vi "Data Access.vi"(8 "error in (no error)":errorcluster, 10 "Data Access Handler":refnum<class "Data Access Handler.lvclass">, 11 "Multi Instrument Batch Msg in":refnum<class "Multi Instrument Batch Msg.lvclass">) -> (0 "error out":errorcluster, 3 "Multi Instrument Batch Msg out":refnum<class "Multi Instrument Batch Msg.lvclass">)   [LabVIEW 2020, in "Instrument Handler.lvlib" / "Multi Instrument Batch Msg.lvclass"]
doc: "Expose class private data to the front panel while letting the Data Access Handler class act on the data."
uses:
  Multi Instrument Batch Msg.lvclass
  C:/Current projects/WS/PPL/HDH.Actor Framework.Core.Msg.lvlibp/Flex Msg/Flex Msg.lvclass
  PPL/HDH.Actor Framework.Core.Msg.lvlibp/Flex Msg/Data Access Handlers/Data Access Handler/Data Access Handler.lvclass
  PPL/HDH.Actor Framework.Core.Publisher.lvlibp/Messages/Response Msg/Response Core/Controls/Ctl_SendFunction.ctl
  PPL/HDH.Actor Framework.Core.Actor.lvlibp/1abvi3w/vi.lib/ActorFramework/Message Enqueuer/Message Priority.ctl
  Multi Instrument Batch Msg.lvclass/Multi Instrument Batch Msg.ctl
  PPL/HDH.Actor Framework.Core.Sequencer.lvlibp/Sequencer Messages/Sequencer Msg/Sequencer Msg.lvclass
  C:/Current projects/WS/PPL/HDH.Actor Framework.Core.Sequencer.lvlibp/Sequencer Messages/Sequencer Msg/Sequencer Msg.lvclass
  PPL/HDH.Actor Framework.Core.Publisher.lvlibp
  PPL/HDH.Actor Framework.Core.Actor.lvlibp/1abvi3w/vi.lib/ActorFramework/Message Enqueuer/Message Enqueuer.lvclass
panel:
  in  "Combined Publish?":bool=TRUE
  in  "Priority":T1=enum."Normal"
  in  "Data Alias Array":string[](array[string])
  in  "Major Data Alias":string
  in  "Publish Data?":bool=TRUE
  in  "Timeout if Waiting":i32=-1
  in  "Send Function":T2=enum."Await Reply"
  in  "Cancel":bool
  in  "OK":bool
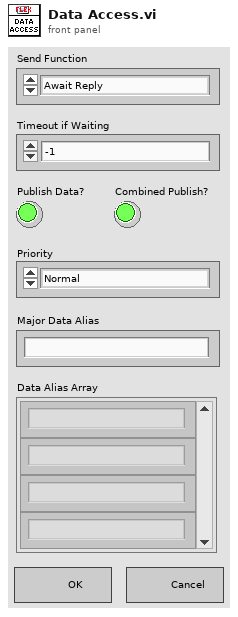
[diagram p1: front panel]
types:
  T1 = typedef "HDH.Actor Framework.Core.Actor.lvlibp/Message Enqueuer.lvclass/Message Priority.ctl" = enum16{"Low", "Normal", "High"}
  T2 = typedef "HDH.Actor Framework.Core.Publisher.lvlibp/Ctl_SendFunction.ctl" = enum16{"Send and Forget", "Request Reply", "Await Reply"}
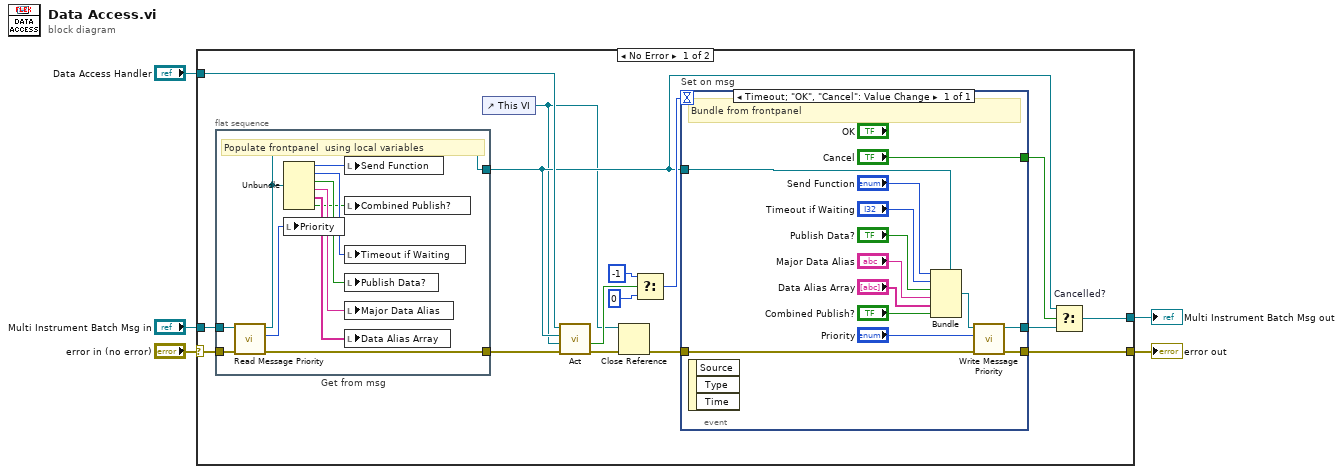
[diagram p0: block diagram]
diagram:
  n1 = case shown="No Error" "error in (no error)" {
    selector: "error in (no error)" -> [w21 w47]
    tunnel: [w14 w47] -> w4
    tunnel: [w9 w46] -> w2
    tunnel: "Multi Instrument Batch Msg in" -> [w12 w46]
    tunnel: "Data Access Handler" -> [w20 _]
    frame No Error {
      n2 = flat-sequence "Get from msg" {
        tunnel: w21 -> [w38]
        tunnel: [w39] -> w7
        tunnel: w12 -> [w40]
        tunnel: [w37] -> w19
        frame #0 {
          # "Populate frontpanel  using local variables"
          n3 = call "Read Message Priority.vi"("error in (no error)"=w38, "Sequencer Msg in"=w40) -> ("error out"=w37:errorcluster, "Priority"=w36:u16, "Sequencer Msg out"=w39:refnum<class "Multi Instrument Batch Msg.lvclass">)  [unwired: 7 in]
          n4 = Unbundle(w39) -> (w45:T2, w44:i32, w43:bool, w42:string, w41:string[], w35:bool)
          n5 = local write "Priority"(w36) -> ()
          n6 = local write "Send Function"(w45) -> ()
          n7 = local write "Combined Publish?"(w35) -> ()
          n8 = local write "Timeout if Waiting"(w44) -> ()
          n9 = local write "Publish Data?"(w43) -> ()
          n10 = local write "Major Data Alias"(w42) -> ()
          n11 = local write "Data Alias Array"(w41) -> ()
        }
      }
      n12 = control-ref of="This VI"() -> (w6:refnum<vi>)
      n13 = call-dynamic "Act.vi"("error in (no error)"=w19, "VI Refnum in"=w6, "Flex Msg type"=w7, "Data Access Handler in"=w20) -> ("error out"=w11:errorcluster, "Await user action?"=w18:bool)  [unwired: 5 in, 1 out]
      n14 = Close Reference(reference=w6, error in (no error)=w11) -> (error out=w13:errorcluster)
      n15 = Select(t=-1, s=w18, f=0 ("t")) -> (s? t:f=w15:i32)
      n16 = event "Set on msg" shown="[0] Timeout;  \"OK\", \"Cancel\": Value Change" {
        selector: _ -> [_]
        dyn-events: _ -> [_]
        timeout: w15 -> [_]
        tunnel: [w24] -> w14
        tunnel: w13 -> [w25]
        tunnel: ["Cancel"] -> w10
        tunnel: [w26] -> w8
        tunnel: w7 -> [w33]
        event Timeout; "OK", "Cancel": Value Change {
          # "Bundle from frontpanel"
          n17 = event-data() -> ()  [unwired: 1 in, 3 out]
          n18 = Bundle(cluster=w33, "Send Function", "Timeout if Waiting", "Publish Data?", "Major Data Alias", "Data Alias Array", "Combined Publish?") -> (w27:refnum<class "Multi Instrument Batch Msg.lvclass">)
          n19 = call "Write Message Priority.vi"("error in (no error)"=w25, "Priority"="Priority", "Sequencer Msg in"=w27) -> ("error out"=w24:errorcluster, "Sequencer Msg out"=w26:refnum<class "Multi Instrument Batch Msg.lvclass">)  [unwired: 7 in]
        }
      }
      n20 = Select "Cancelled?"(t=w7, s=w10, f=w8) -> (s? t:f=w9:refnum<class "Multi Instrument Batch Msg.lvclass">)
    }
    frame Error {
    }
  }
  "error out" <- w4
  "Multi Instrument Batch Msg out" <- w2
